vi "Design a Floating-Point Multirate Filter Part 3.vi"() -> ()   [LabVIEW 2023]
doc: "Part 3 of the Designing a Floating-Point Multirate Filter tutorial."
uses:
  <vilib>/addons/Digital Filter Design/Multirate.llb/DFD MRate Filtering (Wfm).vi
  <vilib>/addons/Digital Filter Design/NI_DigFilterLicensed.lvlib
panel:
  out "Waveform Graph":waveform(dbl)[](graph)
  out "Magnitude Response":cluster{"f0":dbl, "df":dbl, "values":dbl[]}[](graph)
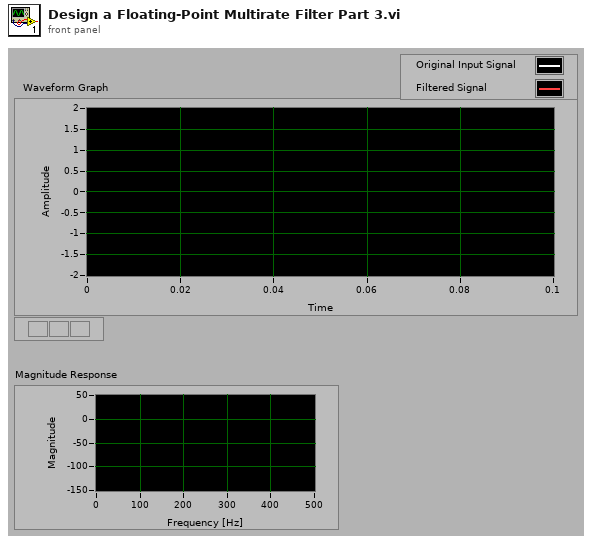
[diagram p1: front panel]
types:
  T1 = typedef "NI_DigFilterLicensed.lvlib/DFD Multirate Filter Obj.ctl" = cluster{"mMRate_Structure":enum16{"CIC", "FIR", "IIR", "Lattice"}, "mMRate_Mode":T2, "mMRate_Factor":i32, "mMRate_FIRParams":cluster{"mMRate_FIR_H":dbl[], "mMRate_FIR_IsNyquist?":bool, "mMRate_FIR_IsSymmetric?":bool}, "mMRate_CICParams":cluster{"mMRate_CIC_#Stage":i32, "mMRate_CIC_Lag":i32, "mMRate_CIC_Type":enum16{"Lowpass", "Highpass"}}, "mMRate_Order":i32, "mMRate_Version":string, "mMRate_Comments":string, "mMRate_RationalFactor":cluster{"mMRate_L":i32, "mMRate_M":i32}, "mMRate_Fs":dbl, "mMRate_Quantized?":bool, "mMRate_QFilterGain":dbl, "mMRate_CoefWl":i16, "mMRate_Scaling":cluster{"mMRate_ScaleByPowerOf2?":bool, "mMRate_ScaleType":T3}, "mMRate_InputWl":i16, "mMRate_OutputWl":i16, "mMRate_OutputMode":T4, "mMRate_MultMode":T5, "mMRate_BitPruning":bool, "mMRate_GainWl":i16, "mMRate_OutputFwl":i16, "mMRate_SumIwl":i16, "mMRate_InputIwl ":i16, "mMRate_SumWl":i16, "mMRate_CoefIwl":i16}
  T2 = typedef "NI_DigFilterLicensed.lvlib/DFD Multirate Mode.ctl" = i16
  T3 = typedef "NI_DigFilterLicensed.lvlib/DFD Coef Norm Type.ctl" = enum16{"No Norm", "Time Domain 1-Norm", "Time Domain 2-Norm", "Time Domain Inf-Norm"}
  T4 = typedef "NI_DigFilterLicensed.lvlib/DFD Round-off Mode.ctl" = enum16{"Nearest", "Truncation"}
  T5 = typedef "NI_DigFilterLicensed.lvlib/DFD FXP MRate Multiply Mode.ctl" = enum16{"Truncated", "Full"}
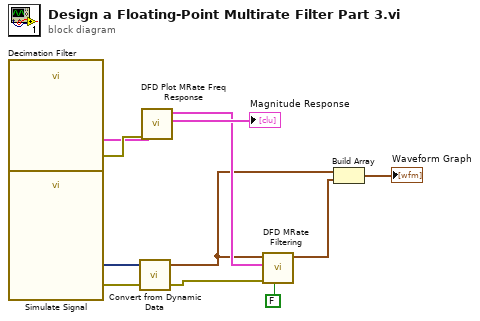
[diagram p0: block diagram]
diagram:
  n1 = call "Decimation Filter"() -> ("error out"=w10:errorcluster, "multirate filter out"=w9:T1)  [unwired: 10 in]
  n2 = call "Simulate Signal"() -> ("Sine with Uniform Noise"=w7:dynamicdata, "error out"=w1:errorcluster)  [unwired: 14 in]
  n3 = call "Convert from Dynamic Data"("Dynamic Data Type"=w7) -> ("Waveform"=w2:waveform(dbl))  [unwired: 3 in]
  n4 = call <vilib>:"DFD Plot MRate Freq Response.vi"("error in (no error)"=w10, "multirate filter in"=w9) -> ("magnitude response"=→"Magnitude Response":cluster{"f0":dbl, "df":dbl, "values":dbl[]}[], "multirate filter out"=w6:T1)  [unwired: 6 in, 2 out]
  n5 = call-poly <vilib>:"DFD MRate Filtering.vi"("zero phase? (T)"=FALSE, "error in (no error)"=w1, "multirate filter"=w6, "signal in"=w2) -> ("signal out"=w5:waveform(dbl))  [unwired: 6 in, 1 out]
  n6 = Build Array "Build Array"(w2, w5) -> (→"Waveform Graph":waveform(dbl)[])
